vi "Clear-reference.vi"(8 "error in (no error)":errorcluster, 10 "Object reference":T1) -> (0 "error out":errorcluster, 3 "Object out":refnum<class "PD-Client.lvclass">)   [LabVIEW 2013, in "PowderDeposition.lvlib" / "PD-Client.lvclass"]
uses:
  PD-Client.lvclass
  Object-reference.ctl
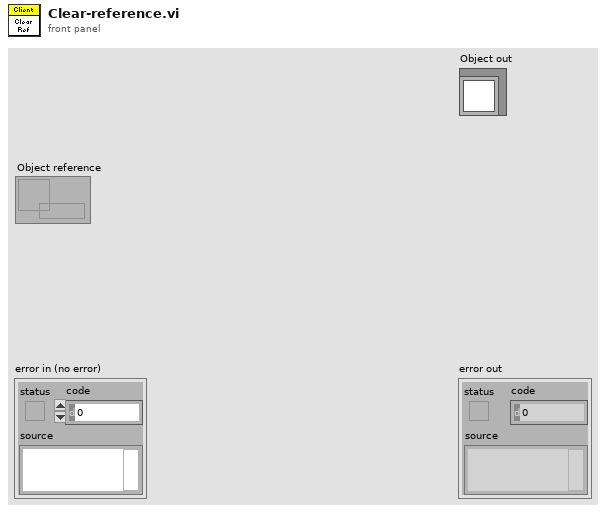
[diagram p1: front panel]
types:
  T1 = typedef "PowderDeposition.lvlib/PD-Client.lvclass/Object-reference.ctl" = refnum<data-value>
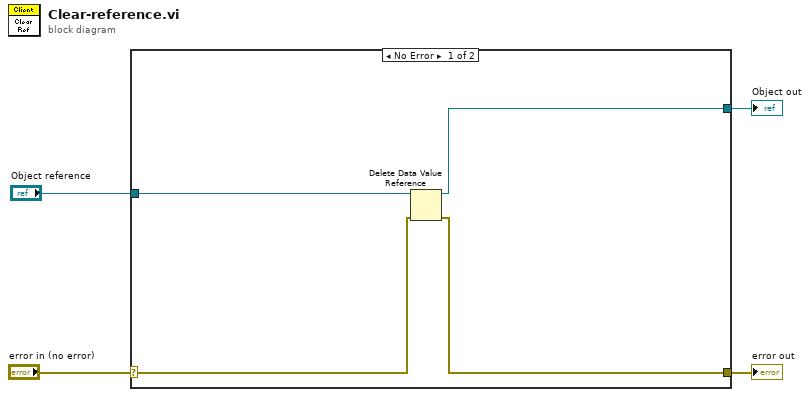
[diagram p0: block diagram]
diagram:
  n1 = case shown="No Error" "error in (no error)" {
    selector: "error in (no error)" -> [w7 w9]
    tunnel: [w6 w9] -> w3
    tunnel: [w5 _] -> w2
    tunnel: "Object reference" -> [w8 _]
    frame No Error {
      n2 = Delete Data Value Reference(data value reference=w8, error in=w7) -> (data value=w5:refnum<class "PD-Client.lvclass">, error out=w6:errorcluster)
    }
    frame Error {
    }
  }
  "error out" <- w3
  "Object out" <- w2
